vi "FPGAcode2_remake.vi"   [LabVIEW 2015]
uses:
  <vilib>/Platform/TimedLoop/XDataNode/timing_clust.ctl
  <vilib>/Platform/TimedLoop/XDataNode/nitl_modes.ctl
  <vilib>/Platform/TimedLoop/XDataNode/wakeup.ctl
  <vilib>/rvi/Emulation/niFpgaSctlEmulationGetInTimedLoop.vi
  <vilib>/rvi/Emulation/niFpgaEmulationReportErrorSimple.vi
  <vilib>/rvi/Emulation/niFpgaGetClockAttributes.vi
  <vilib>/rvi/Emulation/niFpgaCriticalErrorInLSC.vi
  <vilib>/Platform/TimedLoop/XDataNode/XDataNode.xnode
  <vilib>/Platform/TimedLoop/XDataNode/XDNodeRunTimeDep.lvlib
types:
  T1 = typedef "XDNodeRunTimeDep.lvlib/timing_clust.ctl" = cluster{"Expected End [f-1]":u64, "Actual End [f-1]":u64, "Finished Late? [f-1]":bool, "Expected End [i-1]":u64, "Actual End [i-1]":u64, "Finished Late? [i-1]":bool, "Expected Start [i]":u64, "Actual Start [i]":u64, "Expected Start [f]":u64, "Actual Start [f]":u64, "Source Name":string, "Structure Name":string, "Period":i64, "Deadline":i64, "Offset":i64, "Start":i64, "Priority":i32, "Timeout":i32, "Mode":T2, "Wakeup Reason":T3, "Error":errorcluster, "Source Type":string, "Secondary Source Type":string, "Global End Time":u64, "Global Start Time":u64, "Frame Duration":u64, "Iteration Duration":u64, "Assigned CPU":i32, "I/O Scan Engine Mode":u32}
  T2 = typedef "XDNodeRunTimeDep.lvlib/nitl_modes.ctl" = enum32{"No Change", "Process missed periods, maintain original phase", "Discard missed periods, maintain original phase", "Process missed periods, ignore original phase", "Discard missed periods, ignore original phase"}
  T3 = typedef "XDNodeRunTimeDep.lvlib/wakeup.ctl" = enum32{"Normal", "Aborted", "Asynchronous wakeup", "Timing source error", "Timed loop error", "Timeout"}
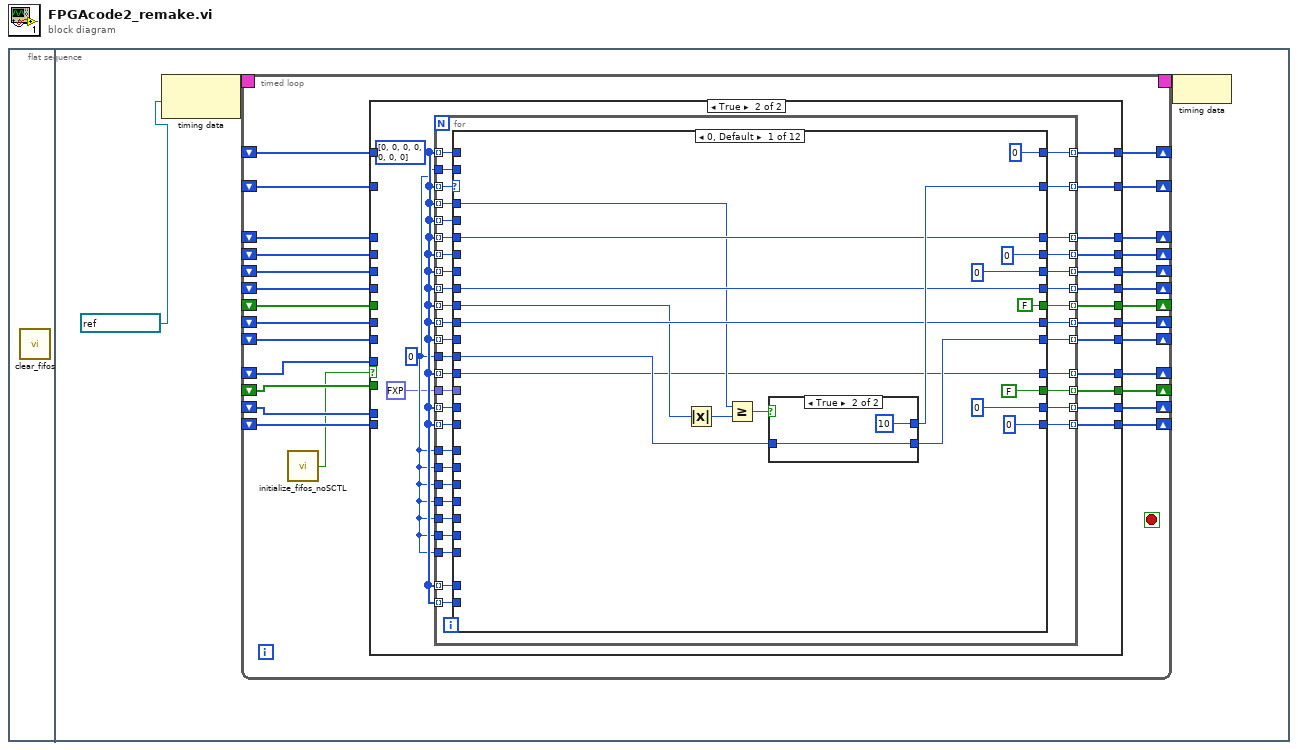
[diagram p0: block diagram]
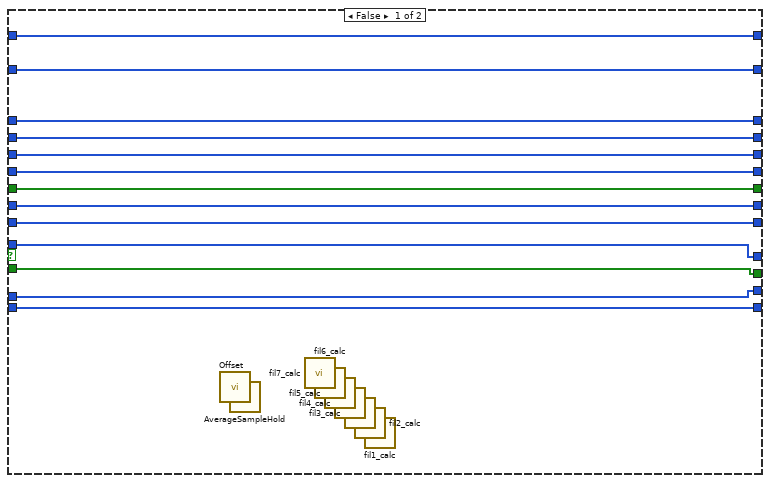
[diagram p2: hidden frame]
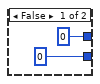
[diagram p3: hidden frame]
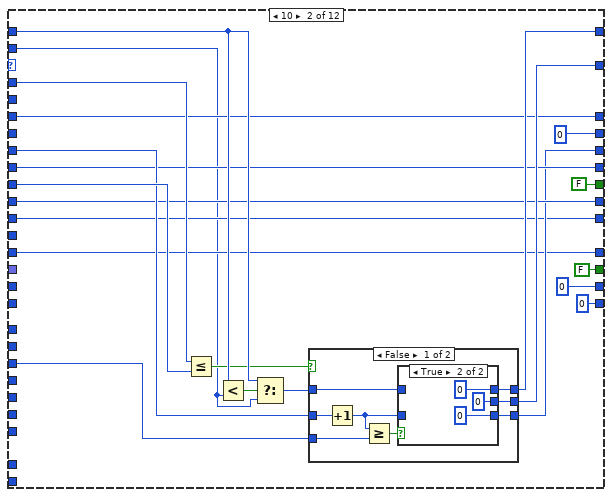
[diagram p4: hidden frame]
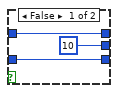
[diagram p5: hidden frame]
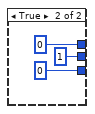
[diagram p6: hidden frame]
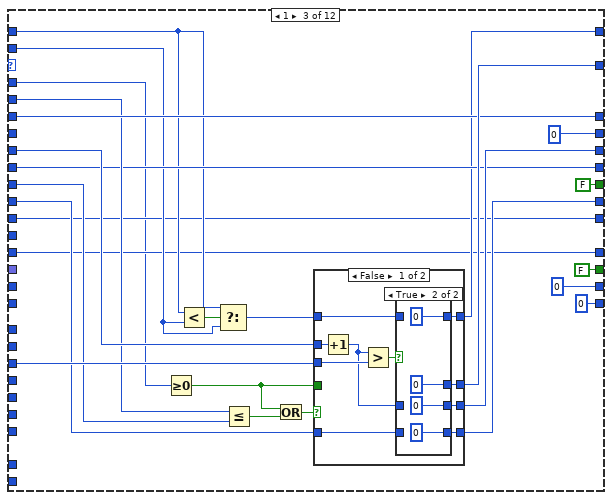
[diagram p7: hidden frame]
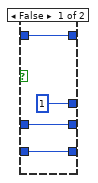
[diagram p8: hidden frame]
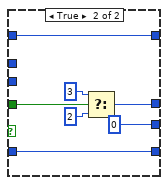
[diagram p9: hidden frame]
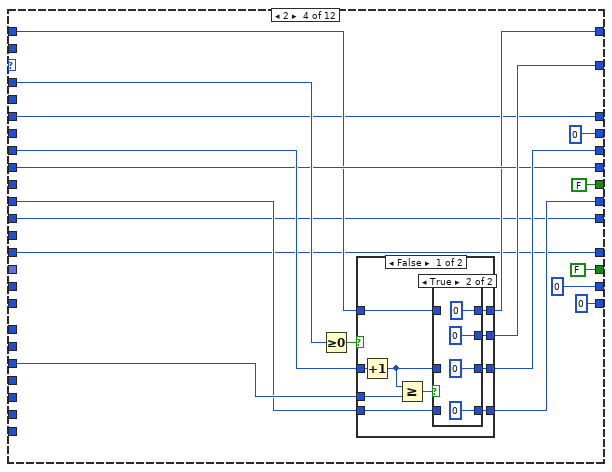
[diagram p10: hidden frame]
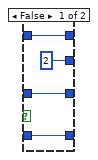
[diagram p11: hidden frame]
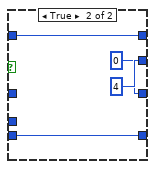
[diagram p12: hidden frame]
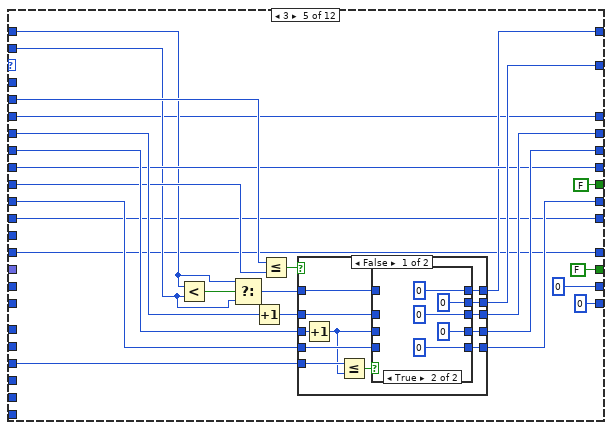
[diagram p13: hidden frame]
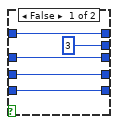
[diagram p14: hidden frame]
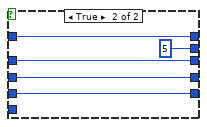
[diagram p15: hidden frame]
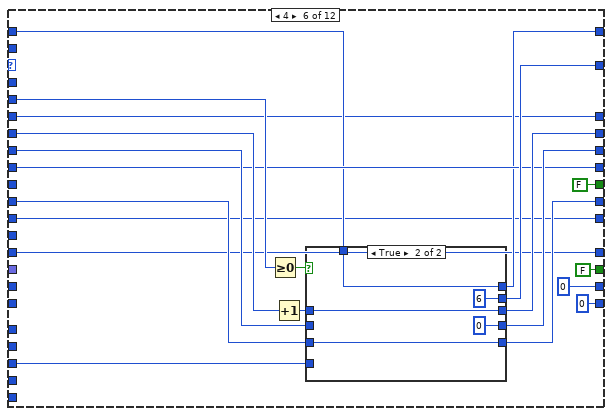
[diagram p16: hidden frame]
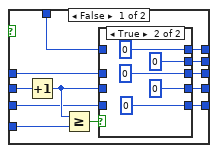
[diagram p17: hidden frame]
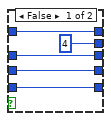
[diagram p18: hidden frame]
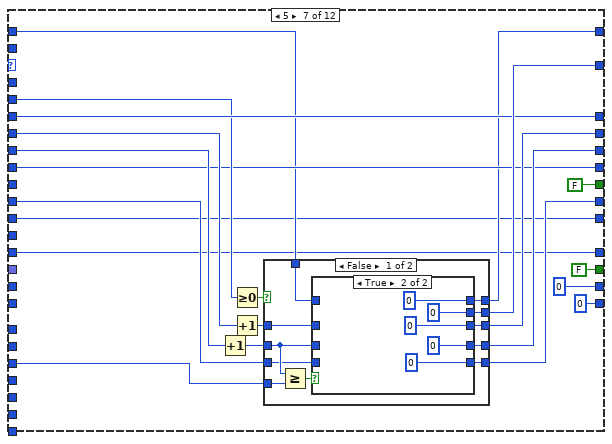
[diagram p19: hidden frame]
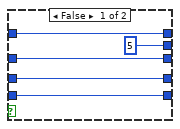
[diagram p20: hidden frame]
diagram:
  n1 = flat-sequence {
    frame #0 {
      n2 = call "clear_fifos.vi"() -> ()  [unwired: 1 in]
    }
    frame #1 {
      n3 = node-c288(refnum<k21> "26.67MHz" ("Source Name")) -> (w3:T1)
      n4 = timed-loop {
        timing: w3 -> [_]
        timing-out: [_] -> w2
        shift-right: [w30] -> _
        shift-left: _ -> [w17]
        shift-right: [w29] -> _
        shift-left: _ -> [w16]
        shift-right: [w28] -> _
        shift-left: _ -> [w15]
        shift-right: [w27] -> _
        shift-left: _ -> [w14]
        shift-right: [w26] -> _
        shift-left: _ -> [w13]
        shift-right: [w25] -> _
        shift-left: _ -> [w12]
        shift-right: [w24] -> _
        shift-left: _ -> [w11]
        shift-right: [w23] -> _
        shift-left: _ -> [w10]
        shift-right: [w22] -> _
        shift-left: _ -> [w9]
        shift-right: [w21] -> _
        shift-left: _ -> [w8]
        shift-right: [w20] -> _
        shift-left: _ -> [w7]
        shift-right: [w19] -> _
        shift-left: _ -> [w6]
        shift-right: [w18] -> _
        shift-left: _ -> [w5]
        stop <- _ stop-if-true
        n5 = call "initialize_fifos_noSCTL.vi"() -> ("Output State"=w4:bool)
        n6 = case shown="True" w4 {
          tunnel: [w43 w56] -> w30
          tunnel: [w42 w55] -> w29
          tunnel: [w41 w54] -> w28
          tunnel: [w40 w53] -> w27
          tunnel: [w39 w52] -> w26
          tunnel: [w38 w51] -> w25
          tunnel: [w37 w50] -> w24
          tunnel: [w36 w49] -> w23
          tunnel: [w35 w48] -> w22
          tunnel: [w34 w47] -> w21
          tunnel: [w33 w46] -> w20
          tunnel: [w32 w45] -> w19
          tunnel: [w31 w44] -> w18
          tunnel: w17 -> [w43 _]
          tunnel: w16 -> [w42 _]
          tunnel: w15 -> [w41 _]
          tunnel: w14 -> [w40 _]
          tunnel: w13 -> [w39 _]
          tunnel: w12 -> [w38 _]
          tunnel: w11 -> [w37 _]
          tunnel: w10 -> [w36 _]
          tunnel: w9 -> [w35 _]
          tunnel: w8 -> [w34 _]
          tunnel: w7 -> [w33 _]
          tunnel: w6 -> [w32 _]
          tunnel: w5 -> [w31 _]
          frame False {
            n7 = call "Offset.vi"() -> ()  [unwired: 11 in, 1 out]
            n8 = call "AverageSampleHold.vi"() -> ()  [unwired: 11 in, 1 out]
            n9 = call "fil7_calc.vi"() -> ()  [unwired: 8 in, 2 out]
            n10 = call "fil6_calc.vi"() -> ()  [unwired: 8 in, 2 out]
            n11 = call "fil5_calc.vi"() -> ()  [unwired: 8 in, 2 out]
            n12 = call "fil4_calc.vi"() -> ()  [unwired: 8 in, 2 out]
            n13 = call "fil3_calc.vi"() -> ()  [unwired: 8 in, 2 out]
            n14 = call "fil2_calc.vi"() -> ()  [unwired: 8 in, 2 out]
            n15 = call "fil1_calc.vi"() -> ()  [unwired: 8 in, 2 out]
          }
          frame True {
            w58 = i16 0 ("Output New Average")
            w59 = i32[] [0, 0, 0, 0, 0, 0, 0]
            n16 = for {
              tunnel: w59 -> [w95] mode=indexing
              tunnel: w59 -> [w94] mode=indexing
              tunnel: w59 -> [w98] mode=indexing
              tunnel: [w79] -> w56 mode=indexing
              tunnel: w59 -> [w96] mode=indexing
              tunnel: [w78] -> w55 mode=indexing
              tunnel: w59 -> [w93] mode=indexing
              tunnel: w59 -> [w82] mode=indexing
              tunnel: [w67] -> w44 mode=indexing
              tunnel: w59 -> [w83] mode=indexing
              tunnel: [w68] -> w45 mode=indexing
              tunnel: w59 -> [w92] mode=indexing
              tunnel: w59 -> [w91] mode=indexing
              tunnel: w59 -> [w85] mode=indexing
              tunnel: w59 -> [w90] mode=indexing
              tunnel: w59 -> [w89] mode=indexing
              tunnel: w59 -> [w88] mode=indexing
              tunnel: w59 -> [w87] mode=indexing
              tunnel: [w77] -> w54 mode=indexing
              tunnel: [w76] -> w53 mode=indexing
              tunnel: [w75] -> w52 mode=indexing
              tunnel: [w74] -> w51 mode=indexing
              tunnel: [w71] -> w49 mode=indexing
              tunnel: [w70] -> w48 mode=indexing
              tunnel: [w69] -> w47 mode=indexing
              tunnel: [w73] -> w50 mode=indexing
              tunnel: [w72] -> w46 mode=indexing
              tunnel: fxp<+,16,7> 0.0 ("Mult1") -> [w84]
              tunnel: w58 -> [w97]
              tunnel: w58 -> [w86]
              tunnel: w59 -> [w81] mode=indexing
              tunnel: w59 -> [w80] mode=indexing
              tunnel: w58 -> [w66]
              tunnel: w58 -> [w65]
              tunnel: w58 -> [w64]
              tunnel: w58 -> [w63]
              tunnel: w58 -> [w62]
              tunnel: w58 -> [w61]
              tunnel: w58 -> [w60]
              n17 = case shown="0, Default" w96 {
                tunnel: w95 -> [w109 w140 w160 w225 _ _ _ _ _ _ _ _]
                tunnel: w94 -> [_ _ w177 _ w268 w316 w363 _ _ _ _ _]
                tunnel: w89 -> [w107 w139 w176 _ w267 _ _ _ _ _ _ _]
                tunnel: w92 -> [_ _ _ _ w270 w324 w372 w415 w472 w501 w531 _]
                tunnel: [0 0 0 0 w276 w322 w365 w400 w471 w499 w529 0] -> w76
                tunnel: [w116 w137 w185 w229 w275 w319 w368 w420 w470 w500 w530 w555] -> w78
                tunnel: w93 -> [w113 w132 w178 w216 w256 w308 w364 w421 w446 w485 w527 w546]
                tunnel: w62 -> [_ w135 w184 w228 w273 w317 w369 _ _ _ _ _]
                tunnel: w91 -> [_ w136 w183 w227 w274 w318 w371 _ _ _ _ _]
                tunnel: [u32 0 w127 w182 w226 w272 w320 w367 u32 0 u32 0 ("Timeout Count in") u32 0 ("Timeout Count in") u32 0 u32 0 ("Timeout Count in")] -> w75
                tunnel: w64 -> [_ _ _ _ _ _ _ _ w469 _ _ _]
                tunnel: w63 -> [_ _ _ _ _ _ _ _ w468 _ _ _]
                tunnel: [w113 w132 w178 w216 w256 w308 w364 w422 w446 w485 w527 w546] -> w77
                tunnel: w61 -> [_ _ _ _ _ _ _ _ w467 _ _ _]
                tunnel: w60 -> [_ _ _ _ _ _ _ _ w466 _ _ _]
                tunnel: w88 -> [w112 w129 w175 w223 w266 w311 w362 w418 w465 w497 w525 _]
                tunnel: [w112 w129 w174 w222 w265 w315 w361 w419 w464 w497 w526 0 ("Noise Level")] -> w71
                tunnel: w90 -> [w111 w130 w173 w221 w264 w314 w360 w417 w447 w493 w522 w548]
                tunnel: [w111 w130 w173 w221 w264 w314 w360 w417 w447 w494 w522 w548] -> w74
                tunnel: [0 ("Old Average In") w133 w172 w220 w263 w313 w359 w416 w460 w490 0 ("Old Average In") 0 ("Old Average In")] -> w79
                tunnel: w81 -> [_ _ _ _ _ _ _ w402 _ _ _ _]
                tunnel: w80 -> [_ _ _ _ _ _ _ w401 _ _ _ _]
                tunnel: [FALSE FALSE ("Data") FALSE FALSE FALSE FALSE FALSE FALSE FALSE ("Data") w484 w516 FALSE ("Data")] -> w73
                tunnel: w98 -> [_ w141 w169 w218 w260 w310 w357 w412 w460 w490 _ _]
                tunnel: w97 -> [_ w121 w168 _ w259 _ _ _ _ _ _ _]
                tunnel: w87 -> [_ w126 w166 w217 w257 w309 w356 w411 w461 w489 _ _]
                tunnel: w86 -> [w104 _ _ _ _ _ _ _ _ _ _ _]
                tunnel: [w105 w126 w166 w217 w257 w309 w356 w411 w461 w489 0 ("Offset") 0 ("Offset")] -> w70
                tunnel: [w103 w125 w165 w215 w255 w307 w355 w410 w448 w495 w520 w553] -> w69
                tunnel: w85 -> [w103 w125 w165 w215 w255 w307 w355 w410 w448 w496 w520 w553]
                tunnel: w65 -> [_ _ _ _ _ _ _ _ w459 _ _ _]
                tunnel: w66 -> [_ _ _ _ _ _ _ _ w458 _ _ _]
                tunnel: w83 -> [_ _ _ _ _ _ _ _ w454 w488 w519 w544]
                tunnel: [0 0 0 0 0 0 0 w406 w453 w486 w514 w541] -> w67
                tunnel: [FALSE FALSE FALSE FALSE FALSE FALSE FALSE FALSE FALSE w483 w515 w545] -> w72
                tunnel: [u16 0 u16 0 u16 0 u16 0 u16 0 u16 0 u16 0 u16 0 u16 0 u16 0 w518 w554] -> w68
                tunnel: w82 -> [_ _ _ _ _ _ _ _ _ _ _ w542]
                tunnel: w84 -> [_ _ _ _ _ _ _ w405 _ _ _ _]
                frame 0, Default {
                  n18 = Absolute Value(x=w107) -> (abs(x)=w106:i32)
                  n19 = Greater Or Equal?(x=w109, y=w106) -> (x >= y?=w114:bool)
                  n20 = case shown="True" w114 {
                    tunnel: [u8 0 u8 10] -> w116
                    tunnel: [0 w119] -> w105
                    tunnel: w104 -> [_ w119]
                    frame False {
                    }
                    frame True {
                    }
                  }
                }
                frame 10 {
                  n21 = Less Or Equal?(x=w140, y=w139) -> (x <= y?=w138:bool)
                  n22 = Less?(x=w141, y=w121) -> (x < y?=w142:bool)
                  n23 = Select(t=w141, s=w142, f=w121) -> (s? t:f=w134:i32)
                  n24 = case shown="False" w138 {
                    tunnel: [w148 u8 1] -> w137
                    tunnel: w136 -> [w145 _]
                    tunnel: w135 -> [w150 _]
                    tunnel: w134 -> [w147 _]
                    tunnel: [w146 0 ("New Average")] -> w133
                    tunnel: [w143 0] -> w127
                    frame False {
                      n25 = Increment(x=w145) -> (x+1=w144:i32)
                      n26 = Greater Or Equal?(x=w144, y=w150) -> (x >= y?=w149:bool)
                      n27 = case shown="True" w149 {
                        tunnel: [u8 10 u8 0] -> w148
                        tunnel: w147 -> [w153 _]
                        tunnel: [w153 0 ("New Average")] -> w146
                        tunnel: w144 -> [w151 _]
                        tunnel: [w151 0] -> w143
                        frame False {
                        }
                        frame True {
                        }
                      }
                    }
                    frame True {
                    }
                  }
                }
                frame 1 {
                  n28 = Greater Or Equal To 0?(x=w160) -> (x >= 0?=w180:bool)
                  n29 = Less?(x=w169, y=w168) -> (x < y?=w170:bool)
                  n30 = Select(t=w169, s=w170, f=w168) -> (s? t:f=w167:i32)
                  n31 = Less Or Equal?(x=w177, y=w176) -> (x <= y?=w179:bool)
                  n32 = Or(x=w180, y=w179) -> (x .or. y?=w181:bool)
                  n33 = case shown="False" w181 {
                    tunnel: [w193 w204] -> w185
                    tunnel: w184 -> [w195 _]
                    tunnel: w183 -> [w192 _]
                    tunnel: [w191 u32 0] -> w182
                    tunnel: w180 -> [_ w205]
                    tunnel: w175 -> [w190 w209]
                    tunnel: [w189 w209] -> w174
                    tunnel: [w188 w210] -> w172
                    tunnel: w167 -> [w186 w210]
                    frame False {
                      n34 = Increment(x=w192) -> (x+1=w187:i32)
                      n35 = Greater?(x=w187, y=w195) -> (0:w194:bool)
                      n36 = case shown="True" w194 {
                        tunnel: [u8 1 u8 0 ("Old Average In")] -> w193
                        tunnel: w187 -> [w198 _]
                        tunnel: [w198 u32 0 ("Old Average In")] -> w191
                        tunnel: w190 -> [w197 _]
                        tunnel: [w197 0 ("Old Average In")] -> w189
                        tunnel: [w196 0 ("Old Average In")] -> w188
                        tunnel: w186 -> [w196 _]
                        frame False {
                        }
                        frame True {
                        }
                      }
                    }
                    frame True {
                      n37 = Select(t=u8 3, s=w205, f=u8 2) -> (s? t:f=w204:u8)
                    }
                  }
                }
                frame 2 {
                  n38 = Greater Or Equal To 0?(x=w225) -> (x >= 0?=w224:bool)
                  n39 = case shown="False" w224 {
                    tunnel: [w238 u8 4] -> w229
                    tunnel: w228 -> [w237 _]
                    tunnel: w227 -> [w235 _]
                    tunnel: [w236 u32 0] -> w226
                    tunnel: w223 -> [w234 w249]
                    tunnel: [w233 w249] -> w222
                    tunnel: [w232 w248] -> w220
                    tunnel: w218 -> [w231 w248]
                    frame False {
                      n40 = Increment(x=w235) -> (x+1=w230:i32)
                      n41 = Greater Or Equal?(x=w230, y=w237) -> (x >= y?=w239:bool)
                      n42 = case shown="True" w239 {
                        tunnel: [u8 2 u8 0] -> w238
                        tunnel: w230 -> [w243 _]
                        tunnel: [w243 u32 0] -> w236
                        tunnel: w234 -> [w241 _]
                        tunnel: [w241 0 ("High Correlation In")] -> w233
                        tunnel: [w240 0 ("Old Average In")] -> w232
                        tunnel: w231 -> [w240 _]
                        frame False {
                        }
                        frame True {
                        }
                      }
                    }
                    frame True {
                    }
                  }
                }
                frame 3 {
                  n43 = Less?(x=w260, y=w259) -> (x < y?=w261:bool)
                  n44 = Select(t=w260, s=w261, f=w259) -> (s? t:f=w258:i32)
                  n45 = Increment(x=w270) -> (x+1=w269:i32)
                  n46 = Less Or Equal?(x=w268, y=w267) -> (x <= y?=w271:bool)
                  n47 = case shown="False" w271 {
                    tunnel: w269 -> [w284 w303]
                    tunnel: [w283 w303] -> w276
                    tunnel: [w286 u8 5] -> w275
                    tunnel: w274 -> [w282 w299]
                    tunnel: w273 -> [w288 _]
                    tunnel: [w285 w299] -> w272
                    tunnel: w266 -> [w281 w301]
                    tunnel: [w280 w301] -> w265
                    tunnel: [w279 w300] -> w263
                    tunnel: w258 -> [w278 w300]
                    frame False {
                      n48 = Increment(x=w282) -> (x+1=w277:i32)
                      n49 = Less Or Equal?(x=w288, y=w277) -> (x <= y?=w287:bool)
                      n50 = case shown="True" w287 {
                        tunnel: [u8 3 u8 0] -> w286
                        tunnel: w277 -> [w292 _]
                        tunnel: [w292 u32 0] -> w285
                        tunnel: w284 -> [w291 _]
                        tunnel: [w291 0] -> w283
                        tunnel: w281 -> [w290 _]
                        tunnel: [w290 0 ("High Correlation In")] -> w280
                        tunnel: [w289 0 ("Old Average In")] -> w279
                        tunnel: w278 -> [w289 _]
                        frame False {
                        }
                        frame True {
                        }
                      }
                    }
                    frame True {
                    }
                  }
                }
                frame 4 {
                  n51 = Greater Or Equal To 0?(x=w316) -> (x >= 0?=w323:bool)
                  n52 = Increment(x=w324) -> (x+1=w321:i32)
                  n53 = case shown="True" w323 {
                    tunnel: [w329 w351] -> w322
                    tunnel: w321 -> [w330 w351]
                    tunnel: [w332 u32 0] -> w320
                    tunnel: [w334 u8 6] -> w319
                    tunnel: w318 -> [w336 _]
                    tunnel: w317 -> [w331 _]
                    tunnel: w311 -> [w328 w348]
                    tunnel: [w327 w348] -> w315
                    tunnel: [w326 w347] -> w313
                    tunnel: w310 -> [w325 w347]
                    frame False {
                      n54 = Increment(x=w336) -> (x+1=w333:i32)
                      n55 = Greater Or Equal?(x=w333, y=w331) -> (x >= y?=w335:bool)
                      n56 = case shown="True" w335 {
                        tunnel: [u8 4 u8 0] -> w334
                        tunnel: w333 -> [w340 _]
                        tunnel: [w340 u32 0] -> w332
                        tunnel: w330 -> [w339 _]
                        tunnel: [w339 0] -> w329
                        tunnel: w328 -> [w338 _]
                        tunnel: [w338 0 ("High Correlation In")] -> w327
                        tunnel: [w337 0 ("Old Average In")] -> w326
                        tunnel: w325 -> [w337 _]
                        frame False {
                        }
                        frame True {
                        }
                      }
                    }
                    frame True {
                    }
                  }
                }
                frame 5 {
                  n57 = Increment(x=w371) -> (x+1=w370:i32)
                  n58 = Greater Or Equal To 0?(x=w363) -> (x >= 0?=w373:bool)
                  n59 = Increment(x=w372) -> (x+1=w366:i32)
                  n60 = case shown="False" w373 {
                    tunnel: w370 -> [w380 _]
                    tunnel: w369 -> [w384 _]
                    tunnel: [w382 u8 6] -> w368
                    tunnel: [w381 u32 0] -> w367
                    tunnel: w366 -> [w379 w397]
                    tunnel: [w378 w397] -> w365
                    tunnel: w362 -> [w376 w396]
                    tunnel: [w377 w396] -> w361
                    tunnel: [w375 w395] -> w359
                    tunnel: w357 -> [w374 w395]
                    frame False {
                      n61 = Greater Or Equal?(x=w380, y=w384) -> (x >= y?=w383:bool)
                      n62 = case shown="True" w383 {
                        tunnel: [u8 5 u8 0] -> w382
                        tunnel: [w388 u32 0] -> w381
                        tunnel: w380 -> [w388 _]
                        tunnel: w379 -> [w387 _]
                        tunnel: [w387 0] -> w378
                        tunnel: [w386 0 ("High Correlation In")] -> w377
                        tunnel: w376 -> [w386 _]
                        tunnel: [w385 0 ("Old Average In")] -> w375
                        tunnel: w374 -> [w385 _]
                        frame False {
                        }
                        frame True {
                        }
                      }
                    }
                    frame True {
                    }
                  }
                }
                frame 6 {
                  n63 = Less?(x=w415, y=w402) -> (x < y?=w404:bool)
                  n64 = Greater Or Equal?(x=w415, y=w401) -> (x >= y?=w403:bool)
                  n65 = And(x=w404, y=w403) -> (x .and. y?=w414:bool)
                  n66 = case shown="True" w414 {
                    tunnel: [0 w432] -> w400
                    tunnel: w415 -> [_ w431]
                    tunnel: [w428 w431] -> w422
                    tunnel: w421 -> [w428 _]
                    tunnel: [u8 0 u8 7] -> w420
                    tunnel: [0 ("High Correlation In") w436] -> w419
                    tunnel: w418 -> [_ w436]
                    tunnel: [0 ("Old Average In") w435] -> w416
                    tunnel: w412 -> [_ w435]
                    frame False {
                    }
                    frame True {
                      n67 = Multiply(x=w431, y=fxp<+,6,1> 1.40625) -> (x*y=w430:fxp<+/-,38,33>)
                      n68 = To Long Integer(number=w430) -> (32bit integer=w429:i32)
                      n69 = Subtract(x=w429, y=19) -> (x-y=w432:i32)
                    }
                  }
                  n70 = Multiply(x=w400, y=w405) -> (x*y=w408:fxp<+/-,48,39>)
                  n71 = To Long Integer(number=w408) -> (32bit integer=w406:i32)
                }
                frame 7 {
                  n72 = Square(x=w446) -> (x^2=w442:i32)
                  n73 = Subtract(x=w461, y=w460) -> (x-y=w463:i32)
                  n74 = To Quad Integer(1:w442) -> (0:w455:i64)
                  n75 = Absolute Value(x=w463) -> (abs(x)=w441:i32)
                  n76 = To Quad Integer(1:w441) -> (0:w456:i64)
                  n77 = Greater Or Equal?(x=w466, y=w441) -> (x >= y?=w445:bool)
                  n78 = Less Or Equal?(x=w467, y=w441) -> (x <= y?=w444:bool)
                  n79 = Multiply(x=w456, y=w455) -> (x*y=w457:i64)
                  n80 = Greater Or Equal?(x=w446, y=w468) -> (x >= y?=w443:bool)
                  n81 = Less Or Equal?(x=w446, y=w469) -> (x <= y?=w440:bool)
                  n82 = Less Or Equal?(x=w457, y=w459) -> (x <= y?=w438:bool)
                  n83 = Greater Or Equal?(x=w457, y=w458) -> (x >= y?=w439:bool)
                  n84 = Compound Arithmetic op=AND(w445, w444, w443, w440, w438, w439) -> (w462:bool)
                  n85 = case shown="True" w462 {
                    tunnel: w472 -> [_ w482]
                    tunnel: [0 w480] -> w471
                    tunnel: [u8 0 u8 8] -> w470
                    tunnel: w465 -> [_ w481]
                    tunnel: [0 ("High Correlation In") w481] -> w464
                    tunnel: w454 -> [_ w478]
                    tunnel: [0 w477] -> w453
                    frame False {
                    }
                    frame True {
                      n86 = Decrement(x=w482) -> (x-1=w480:i32)
                      n87 = Decrement(x=w478) -> (x-1=w477:i32)
                    }
                  }
                }
                frame 8 {
                  n88 = Decrement(x=w501) -> (x-1=w502:i32)
                  n89 = Subtract(x=w489, y=w490) -> (x-y=w492:i32)
                  n90 = Less Or Equal To 0?(x=w502) -> (x <= 0?=w484:bool)
                  n91 = Absolute Value(x=w492) -> (abs(x)=w491:i32)
                  n92 = case shown="True" w484 {
                    tunnel: [u8 8 u8 9] -> w500
                    tunnel: [w506 w512] -> w499
                    tunnel: w485 -> [_ w510]
                    tunnel: w502 -> [w506 _]
                    tunnel: w496 -> [w504 _]
                    tunnel: [w504 w510] -> w495
                    tunnel: [w503 w509] -> w494
                    tunnel: w493 -> [w503 _]
                    tunnel: w491 -> [_ w509]
                    frame False {
                    }
                    frame True {
                      n93 = To Fixed-Point(number=w510) -> (fixed-point=w507:fxp<+/-,32,32>)  [unwired: 1 in]
                      n94 = Multiply(x=fxp<+,2,1> 1.5, y=w507) -> (x*y=w513:fxp<+/-,34,33>)
                      n95 = To Long Integer(number=w513) -> (32bit integer=w512:i32)
                    }
                  }
                  n96 = Decrement(x=w488) -> (x-1=w486:i32)
                  n97 = Less Or Equal To 0?(x=w486) -> (x <= 0?=w483:bool)
                }
                frame 9 {
                  n98 = Decrement(x=w531) -> (x-1=w528:i32)
                  n99 = Less Or Equal To 0?(x=w528) -> (x <= 0?=w517:bool)
                  n100 = case shown="True" w517 {
                    tunnel: [w534 0] -> w529
                    tunnel: [u8 9 u8 12] -> w530
                    tunnel: w528 -> [w534 _]
                    tunnel: w525 -> [w533 _]
                    tunnel: [w533 0 ("Noise Level")] -> w526
                    tunnel: [u16 0 u16 550] -> w518
                    frame False {
                    }
                    frame True {
                    }
                  }
                  n101 = Decrement(x=w519) -> (x-1=w514:i32)
                  n102 = Not(x=w517) -> (.not. x?=w516:bool)
                  n103 = Less Or Equal To 0?(x=w514) -> (x <= 0?=w515:bool)
                }
                frame 12 {
                  n104 = Decrement(x=w544) -> (x-1=w540:i32)
                  n105 = Less Or Equal To 0?(x=w540) -> (x <= 0?=w543:bool)
                  n106 = case shown="True" w543 {
                    tunnel: [FALSE w561] -> w545
                    tunnel: [u8 12 w566] -> w555
                    tunnel: w542 -> [w559 w567]
                    tunnel: [w559 w565] -> w554
                    tunnel: [w557 0] -> w541
                    tunnel: w540 -> [w557 _]
                    frame False {
                    }
                    frame True {
                      n107 = Decrement(x=w567) -> (x-1=w564:i32)
                      n108 = Less Or Equal To 0?(x=w564) -> (x <= 0?=w562:bool)
                      n109 = case shown="False" w562 {
                        tunnel: [u8 12 u8 0] -> w566
                        tunnel: [w568 u16 0] -> w565
                        tunnel: w564 -> [w568 _]
                        frame False {
                        }
                        frame True {
                        }
                      }
                      n110 = Not(x=w562) -> (.not. x?=w561:bool)
                    }
                  }
                }
              }
            }
          }
        }
      }
      n111 = node-c288(w2) -> ()
    }
  }
